vi "OP300ZP_SN_Reader.vi"(11 "Fichier txt":string) -> (3 "SN":string)   [LabVIEW 2020]
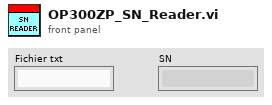
[diagram p1: front panel]
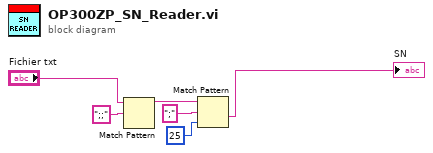
[diagram p0: block diagram]
diagram:
  n1 = Match Pattern(string="Fichier txt", regular expression=";;" ("expression régulière")) -> (before substring=w2:string)  [unwired: 1 in, 3 out]
  n2 = Match Pattern(string=w2, regular expression=";" ("expression régulière"), offset (0)=25) -> (after substring=→"SN":string)  [unwired: 3 out]
